vi "SSL Detection Frame Simple Estimator Kalman VelCmd.vi"(4 "Lado":enum16{"Esquerdo", "Direito"}(ring) caption="Enum", 5 "Last IA State":T1={"our_robots"=[], "enemy_robots"=[], "balls"=[], "geometry"={"line_width"=0, "field_length"=0, "field_width"=0, "boundary_width"=0, "referee_width"=0, "goal_width"=0, "goal_depth"=0, "goal_wall_width"=0, "center_circle_radius"=0, "defense_radius"=0, "defense_stretch"=0, "free_kick_from_defense_dist"=0, "penalty_spot_from_field_line_dist"=0, "penalty_line_from_spot_dist"=0}, "IA Judge"={"stage"="", "command"="", "our_goalie_id"=0.0, "enemy_goalie_id"=0.0, "command enum"=enum."Halt", "Time"=enum."Azul"}, "Received Timestamp"=timestamp(0 s since 1904-01-01), "Events"={"Touch"=FALSE, "Ball out"=FALSE, "id touch"=0.0, "Ball out of \nVision"=FALSE, "Ball inside \nGoalie area"=FALSE, "Robot not responding"=FALSE, "Robots responding status"=[1.0, 1.0, 1.0, 1.0, 1.0, 1.0], "Enemy Ball \nPossession"=FALSE, "Pass State"=FALSE, "id end of pass"=0.0, "Kick"=FALSE, "Id ini Possession"=0.0, "Ball Possesion"=FALSE, "Id Possesion"=0.0, "Direct Kick"=FALSE, "2nd Strk Ativo"=FALSE}}, 6 "Time":enum16{"Azul", "Amarelo"}(ring) caption="Enum", 7 "Enable":bool, 8 "ignora esquerda?":bool=TRUE, 9 "ignora lado?":bool=TRUE, 10 "Field Size":T12, 11 "Detection Frame In":T13 {"robots_blue"."height" format="%+4.3f"; "robots_blue"."pixel_y" format="%+4.3f"; "robots_blue"."pixel_x" format="%+4.3f"; "robots_blue"."orientation" format="%+4.3f"; "robots_blue"."y" format="%+4.3f"; "robots_blue"."confidence" format="%4.3f"; "robots_blue"."x" format="%+4.3f"; "robots_yellow"."height" format="%+4.3f"; "robots_yellow"."pixel_y" format="%+4.3f"; "robots_yellow"."pixel_x" format="%+4.3f"; "robots_yellow"."orientation" format="%+4.3f"; "robots_yellow"."y" format="%+4.3f"; "robots_yellow"."confidence" format="%4.3f"; "robots_yellow"."x" format="%+4.3f"}) -> (2 "Field Size Out":T12, 3 "Detection Frame Out":T13 {"robots_blue"."height" format="%+4.3f"; "robots_blue"."pixel_y" format="%+4.3f"; "robots_blue"."pixel_x" format="%+4.3f"; "robots_blue"."orientation" format="%+4.3f"; "robots_blue"."y" format="%+4.3f"; "robots_blue"."confidence" format="%4.3f"; "robots_blue"."x" format="%+4.3f"; "robots_yellow"."height" format="%+4.3f"; "robots_yellow"."pixel_y" format="%+4.3f"; "robots_yellow"."pixel_x" format="%+4.3f"; "robots_yellow"."orientation" format="%+4.3f"; "robots_yellow"."y" format="%+4.3f"; "robots_yellow"."confidence" format="%4.3f"; "robots_yellow"."x" format="%+4.3f"})   [LabVIEW 2018]
uses:
  SSL Detection Frame.ctl
  SSL Detection Robot.ctl
  <vilib>/Analysis/Matrix/Datatypes/RealMatrix.ctl
  SSL Detection Ball.ctl
  Core/AI Input.ctl
  Core/AI Robot.ctl
  Intel/Functions Enum.ctl
  Intel/AttackerStates.ctl
  Path Planning/RRT/PathDests.ctl
  Path Planning/RRT/PathDest.ctl
  Core/AI Ball.ctl
  Core/Field Size.ctl
  Core/AI Judge.ctl
  Intel/Command Enum.ctl
  Events/Events.ctl
  <vilib>/Analysis/Matrix/NI_Matrix.lvlib
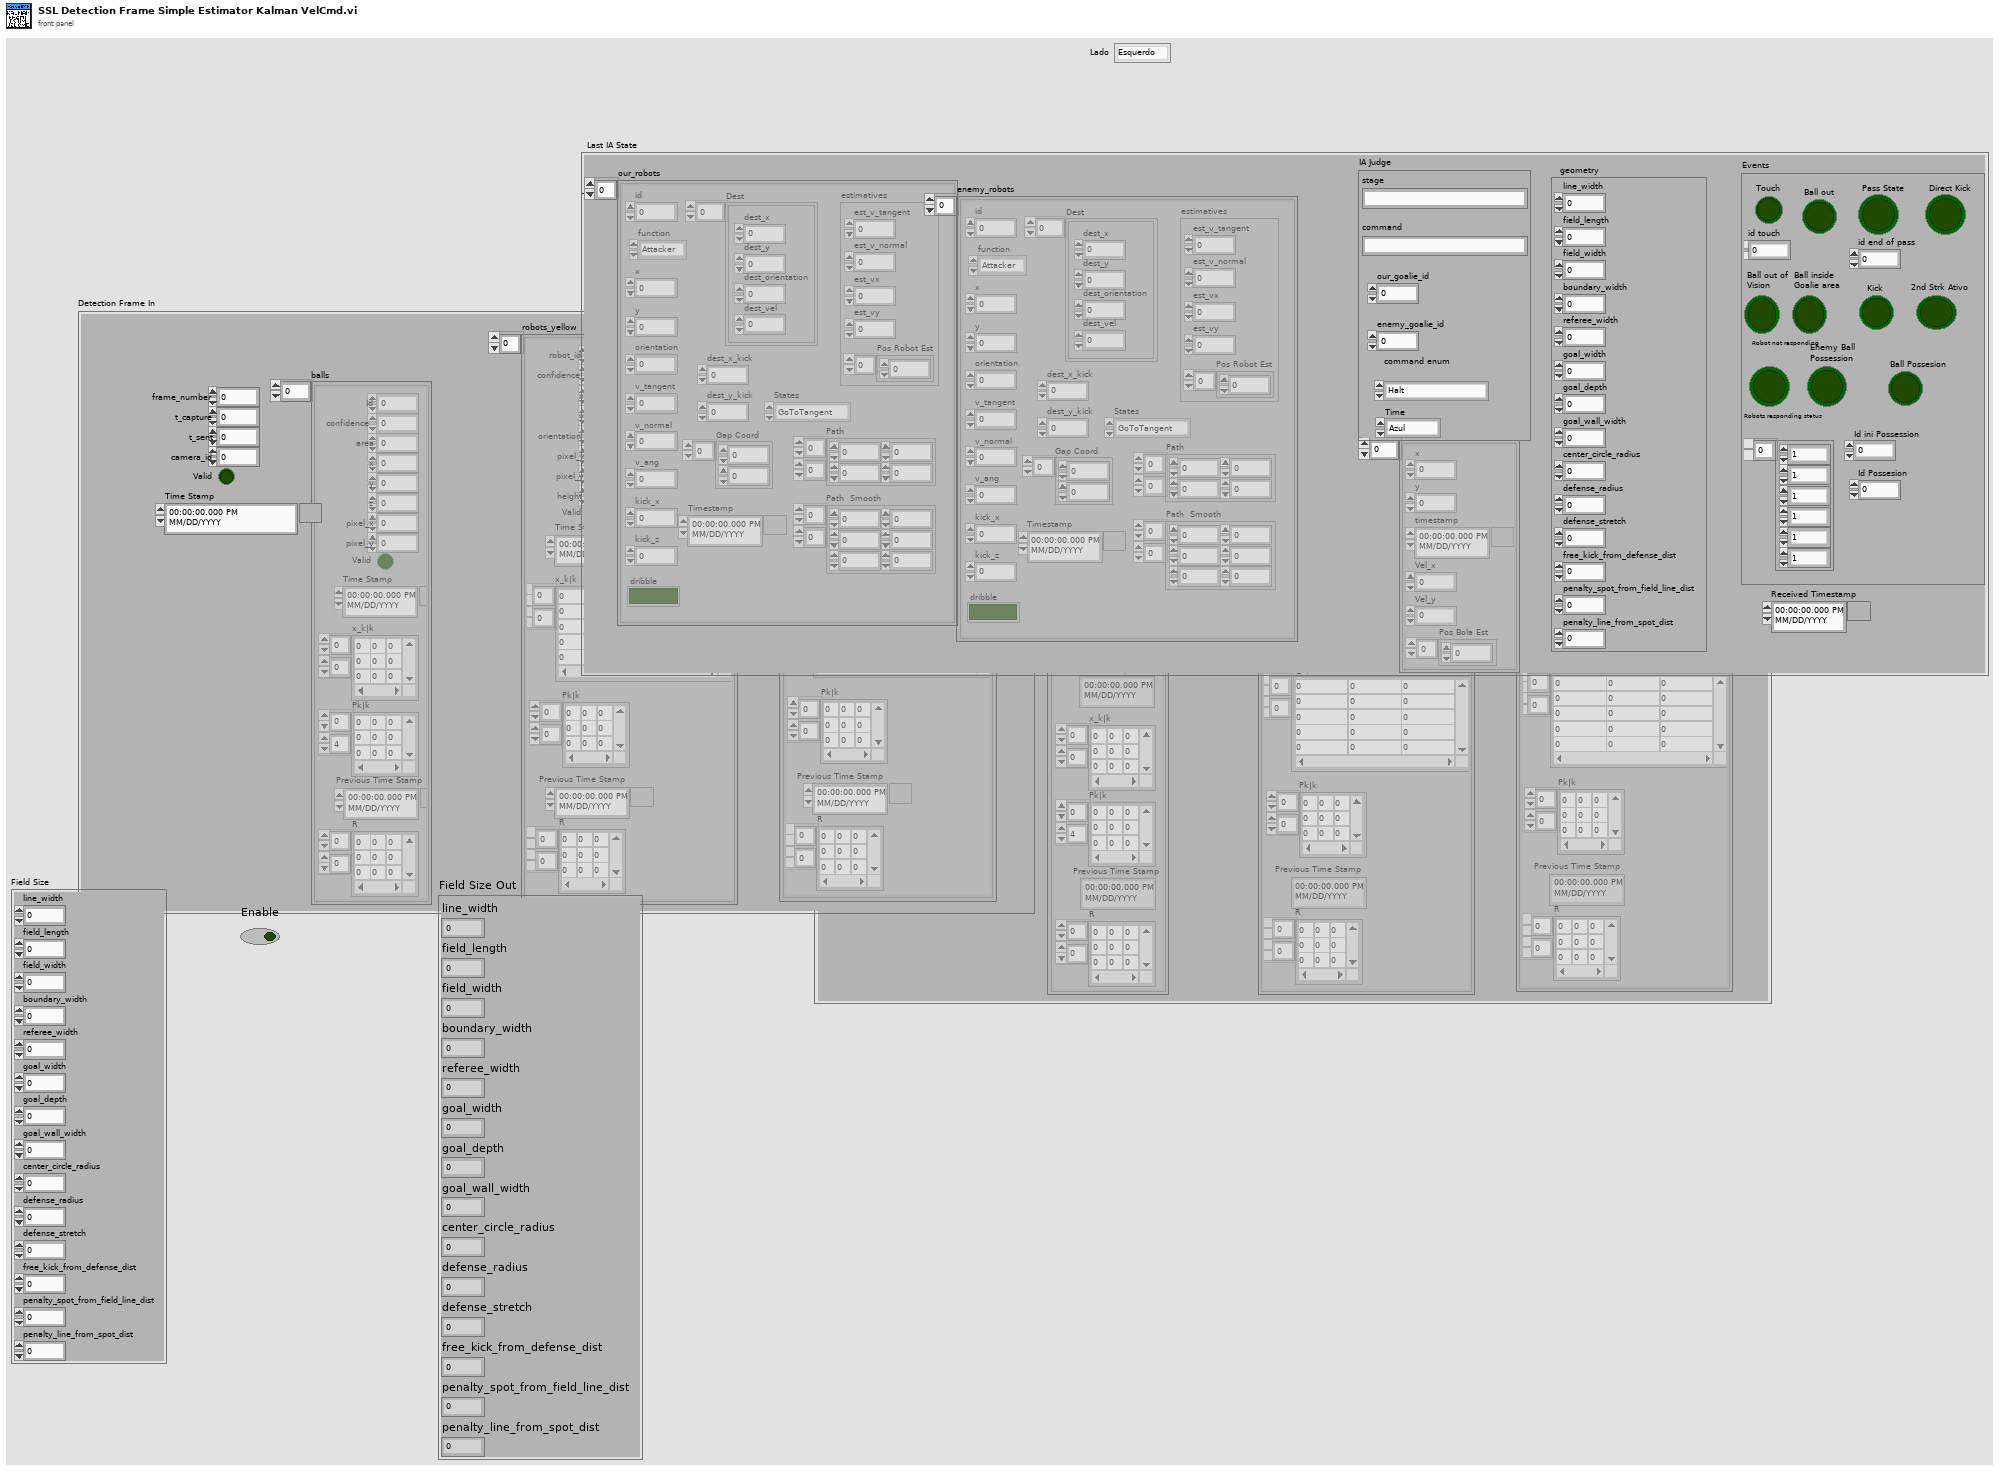
[diagram p1: front panel]
types:
  T1 = typedef "AI Input.ctl" = cluster{"our_robots":T2[], "enemy_robots":T2[], "balls":T7[], "geometry":T8, "IA Judge":T9, "Received Timestamp":timestamp, "Events":T11}
  T2 = typedef "AI Robot.ctl" = cluster{"id":u32, "function":T3, "x":dbl, "y":dbl, "orientation":dbl, "v_tangent":dbl, "v_normal":dbl, "v_ang":dbl, "kick_x":dbl, "kick_z":dbl, "dribble":bool, "Timestamp":timestamp, "estimatives":cluster{"est_v_tangent":dbl, "est_v_normal":dbl, "est_vx":dbl, "est_vy":dbl, "Pos Robot Est":dbl[]}, "dest_x_kick":dbl, "dest_y_kick":dbl, "Gap Coord":dbl[], "States":T4, "Path ":dbl[][], "Path  Smooth":dbl[][], "Dest":T5}
  T3 = typedef "Functions Enum.ctl" = enum16{"2nd Striker", "Attacker", "Goalie", "Defender", "Striker", "Goto 0", "Dummy", "Kicker", "ZigZag 0", "ZigZag 1", "ZigZag 2", "ZigZag 3", "ZigZag 4", "ZigZag 5", "ZigZag 6", "ZigZag 7", "ZigZag 8", ""}
  T4 = typedef "AttackerStates.ctl" = enum16{"Pass", "GoToTangent", "BallGetting", "GoToKick", ""}
  T5 = typedef "PathDests.ctl" = T6[]
  T6 = typedef "PathDest.ctl" = cluster{"dest_x":dbl, "dest_y":dbl, "dest_orientation":dbl, "dest_vel":dbl}
  T7 = typedef "AI Ball.ctl" = cluster{"x":dbl, "y":dbl, "timestamp":timestamp, "Vel_x":dbl, "Vel_y":dbl, "Pos Bola Est":dbl[]}
  T8 = typedef "Field Size.ctl" = cluster{"line_width":u32, "field_length":u32, "field_width":u32, "boundary_width":u32, "referee_width":u32, "goal_width":u32, "goal_depth":u32, "goal_wall_width":u32, "center_circle_radius":u32, "defense_radius":u32, "defense_stretch":u32, "free_kick_from_defense_dist":u32, "penalty_spot_from_field_line_dist":u32, "penalty_line_from_spot_dist":u32}
  T9 = typedef "AI Judge.ctl" = cluster{"stage":string, "command":string, "our_goalie_id":dbl, "enemy_goalie_id":dbl, "command enum":T10, "Time":enum16{"Azul", "Amarelo"}}
  T10 = typedef "Command Enum.ctl" = enum16{"Halt", "Stop", "Force Start", "PKA Normal Start", "Prepare Kickoff Ally", "PKE Normal Start", "Prepare Kickoff Enemy", "Prepare Penalty Ally", "PPA Normal Start", "Prepare Penalty Enemy", "PPE Normal Start", "Direct Free Enemy", "Direct Free Ally", "Indirect Free Enemy", "Indirect Free Ally", "Timeout Enemy", "Timeout Ally", "Goal Enemy", "Goal Ally", "Ball Placement Enemy", "Ball Placement Ally", "Normal Half Time", "Extra Time Break", "Extra Half Time", "None", "Post Game"}
  T11 = typedef "Events.ctl" = cluster{"Touch":bool, "Ball out":bool, "id touch":dbl, "Ball out of \nVision":bool, "Ball inside \nGoalie area":bool, "Robot not responding":bool, "Robots responding status":dbl[], "Enemy Ball \nPossession":bool, "Pass State":bool, "id end of pass":dbl, "Kick":bool, "Id ini Possession":dbl, "Ball Possesion":bool, "Id Possesion":dbl, "Direct Kick":bool, "2nd Strk Ativo":bool}
  T12 = cluster{"line_width":u32, "field_length":u32, "field_width":u32, "boundary_width":u32, "referee_width":u32, "goal_width":u32, "goal_depth":u32, "goal_wall_width":u32, "center_circle_radius":u32, "defense_radius":u32, "defense_stretch":u32, "free_kick_from_defense_dist":u32, "penalty_spot_from_field_line_dist":u32, "penalty_line_from_spot_dist":u32}
  T13 = typedef "SSL Detection Frame.ctl" = cluster{"frame_number":u32, "t_capture":dbl, "t_sent":dbl, "camera_id":u32, "robots_yellow":T14[], "robots_blue":T14[], "balls":T16[], "Valid":bool, "Time Stamp":timestamp}
  T14 = typedef "SSL Detection Robot.ctl" = cluster{"x":sgl, "robot_id":u32, "confidence":sgl, "y":sgl, "orientation":sgl, "pixel_x":sgl, "pixel_y":sgl, "height":sgl, "Valid":bool, "Time Stamp":timestamp, "x_k|k":T15, "Pk|k":T15, "Previous Time Stamp":timestamp, "R":T15}
  T15 = typedef "NI_Matrix.lvlib/RealMatrix.ctl" = dbl[][]
  T16 = typedef "SSL Detection Ball.ctl" = cluster{"x":sgl, "area":u32, "confidence":sgl, "y":sgl, "z":sgl, "pixel_x":sgl, "pixel_y":sgl, "Valid":bool, "Time Stamp":timestamp, "x_k|k":T15, "Pk|k":T15, "Id":u32, "Previous Time Stamp":timestamp, "R":T15}
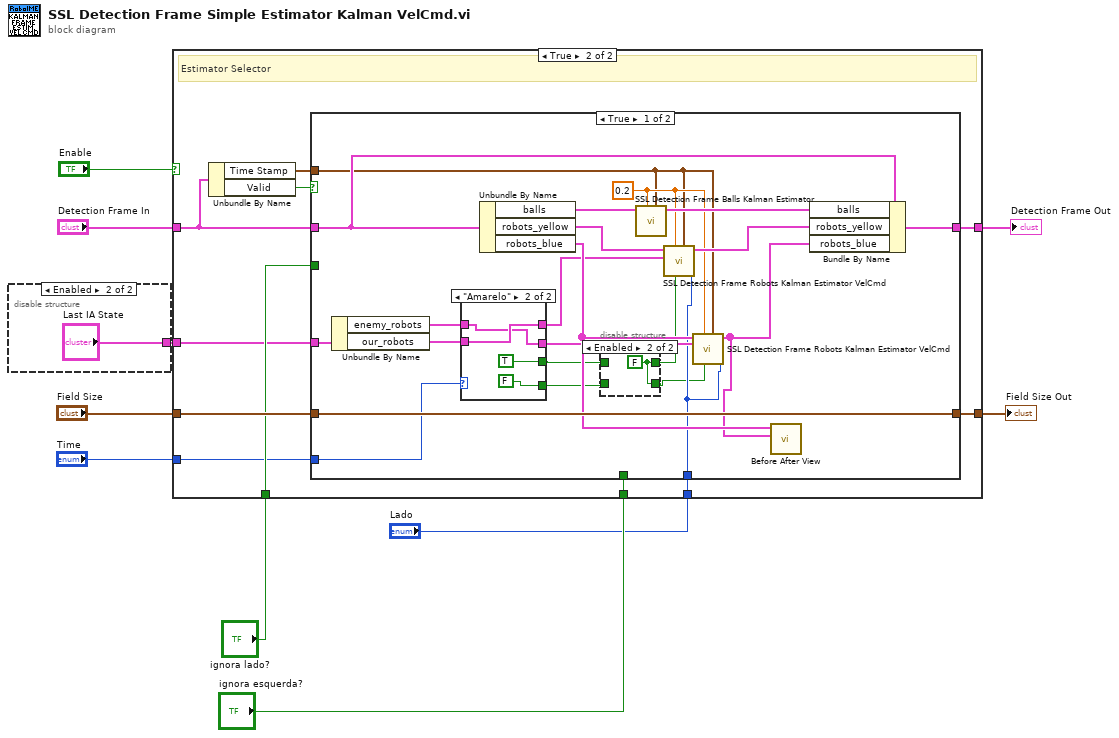
[diagram p0: block diagram]
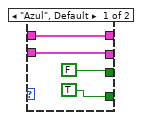
[diagram p5: hidden frame]
diagram:
  n1 = disable-structure shown="Enabled" {
    disable-tunnel: [_ "Last IA State"] -> w3
    frame Disabled {
    }
    frame Enabled {
    }
  }
  n2 = case shown="True" "Enable" {
    tunnel: [w13 w24] -> w10
    tunnel: "Detection Frame In" -> [w13 w21]
    tunnel: "Field Size" -> [w12 w23]
    tunnel: [w12 w22] -> w7
    tunnel: "ignora lado?" -> [_ w18]
    tunnel: "ignora esquerda?" -> [_ w17]
    tunnel: w3 -> [_ w16]
    tunnel: "Time" -> [_ w15]
    tunnel: "Lado" -> [_ w14]
    frame False {
    }
    frame True {
      # "Estimator Selector"
      n3 = Unbundle By Name(w21) -> ("Time Stamp"=w19:timestamp, "Valid"=w20:bool)
      n4 = case shown="True" w20 {
        tunnel: w21 -> [w46 w58]
        tunnel: [w45 w58] -> w24
        tunnel: w19 -> [w29 _]
        tunnel: w23 -> [w42 w59]
        tunnel: [w42 w59] -> w22
        tunnel: w18 -> [_ _]
        tunnel: w17 -> [_ _]
        tunnel: w16 -> [w38 _]
        tunnel: w15 -> [w37 _]
        tunnel: w14 -> [w33 _]
        frame True {
          w30 = 0.2 ("Life Time")
          n5 = Unbundle By Name(w38) -> ("enemy_robots"=w36:T2[], "our_robots"=w35:T2[])
          n6 = case shown="\"Amarelo\"" w37 {
            tunnel: w36 -> [w53 w56]
            tunnel: w35 -> [w52 w57]
            tunnel: [w53 w57] -> w31
            tunnel: [w52 w56] -> w34
            tunnel: [FALSE TRUE] -> w28
            tunnel: [TRUE FALSE] -> w25
            frame "Azul", Default {
            }
            frame "Amarelo" {
            }
          }
          n7 = Unbundle By Name(w46) -> ("balls"=w44:T16[], "robots_yellow"=w32:T14[], "robots_blue"=w41:T14[])
          n8 = disable-structure shown="Enabled" {
            disable-tunnel: w28 -> [w48 _]
            disable-tunnel: [w48 w49] -> w27
            disable-tunnel: [w47 w49] -> w26
            disable-tunnel: w25 -> [w47 _]
            frame Disabled {
            }
            frame Enabled {
              w49 = FALSE
            }
          }
          n9 = call "SSL Detection Frame Balls Kalman Estimator.vi"("Time Stamp 2"=w29, "Life Time 2"=w30, "Detection Ball \nArray"=w44) -> ("balls"=w39:T16[])  [unwired: 8 in]
          n10 = call "SSL Detection Frame Robots Kalman Estimator VelCmd.vi"("Lado"=w33, "Time Stamp"=w29, 6:"our_robots"=w27, "Life Time"=w30, 10:"our_robots"=w31, "Robots"=w32) -> ("Robots Out"=w43:T14[])  [unwired: 5 in]
          n11 = call "SSL Detection Frame Robots Kalman Estimator VelCmd.vi"("Lado"=w33, "Time Stamp"=w29, 6:"our_robots"=w26, "Life Time"=w30, 10:"our_robots"=w34, "Robots"=w41) -> ("Robots Out"=w40:T14[])  [unwired: 5 in]
          n12 = call "Before After View.vi"("after"=w40, "before"=w41) -> ()  [unwired: 10 in]
          n13 = Bundle By Name(cluster=w46, "balls"=w39, "robots_yellow"=w43, "robots_blue"=w40) -> (w45:T13)
        }
        frame False {
        }
      }
    }
  }
  "Detection Frame Out" <- w10
  "Field Size Out" <- w7
